vi "Read Frequency Spectra.vi"(8 "error in (no error)":errorcluster, 10 "data (all)":u16(ring)=2 items=["voltage", "current", "all"], 11 "VI Probe in":refnum<class "PL MKS VI Probe.lvclass">) -> (0 "error out":errorcluster, 2 "spectra":T1, 3 "VI Probe out":refnum<class "PL MKS VI Probe.lvclass">)   [LabVIEW 2015, in "PL MKS VI Probe.lvclass"]
doc: "Reads frequency spectra."
uses:
  PL MKS VI Probe.lvclass
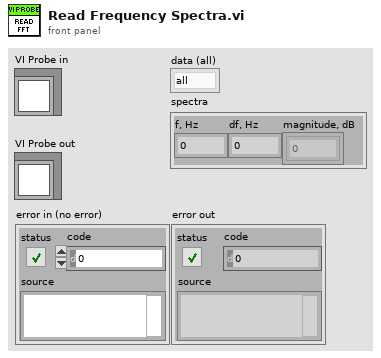
[diagram p1: front panel]
types:
  T1 = cluster{"f, Hz":dbl, "df, Hz":dbl, "magnitude, dB":dbl[][]}
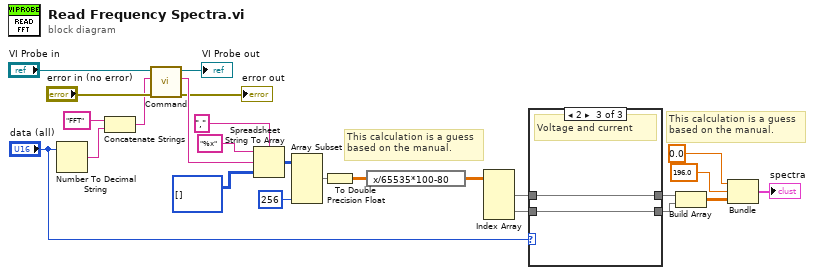
[diagram p0: block diagram]
diagram:
  # "This calculation is a guess\nbased on the manual."
  # "This calculation is a guess\nbased on the manual."
  n1 = Number To Decimal String(number="data (all)") -> (decimal integer string=w22:string)  [unwired: 1 in]
  n2 = Concatenate Strings("FFT" ("format string"), w22) -> (w20:string)
  n3 = call "Command.vi"("error in (no error)"="error in (no error)", "command"=w20, "VI Probe in"="VI Probe in") -> ("error out"=→"error out":errorcluster, "response data"=w16:string, "VI Probe out"=→"VI Probe out":refnum<class "PL MKS VI Probe.lvclass">)  [unwired: 6 in]
  n4 = Spreadsheet String To Array(delimiter (Tab)="," ("format string"), format string="%x", spreadsheet string=w16, array type (2D Dbl)=u16[][] []) -> (array=w12:u16[][])
  n5 = Array Subset(array=w12, length (col)=256 ("length")) -> (w5:u16[][])  [unwired: 3 in]
  n6 = To Double Precision Float(number=w5) -> (double precision float=w6:dbl[][])
  n7 = expression code="x/65535*100-80"(w6) -> (w4:dbl[][])
  n8 = Index Array(array=w4) -> (element #1=w11:dbl[], element #2=w10:dbl[])  [unwired: 4 in]
  n9 = case shown="2" "data (all)" {
    tunnel: w11 -> [w26 w27 w29]
    tunnel: w10 -> [_ _ w28]
    tunnel: [w26 _ w29] -> w3
    tunnel: [_ w27 w28] -> w2
    frame 0, Default {
      # "Voltage"
    }
    frame 1 {
      # "Current"
    }
    frame 2 {
      # "Voltage and current"
    }
  }
  n10 = Build Array(w3, w2) -> (w7:dbl[][])
  n11 = Bundle(0.0, 196.0, w7) -> (→"spectra":cluster{dbl, dbl, dbl[][]})  [unwired: 1 in]
